vi "Create.vi"(8 "error in (no error)":errorcluster, 11 "Session in":refnum<class "Session.lvclass">) -> (0 "error out":errorcluster, 3 "Session out":refnum<class "Session.lvclass">)   [LabVIEW 2020, in "HTTP Server.lvlib" / "Session.lvclass"]
uses:
  Session.lvclass
  Session.lvclass/Session.ctl
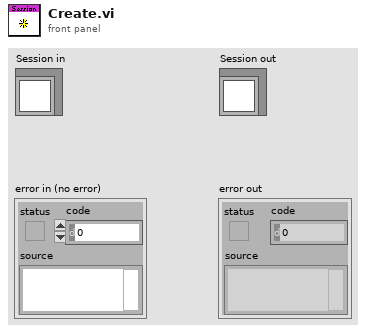
[diagram p1: front panel]
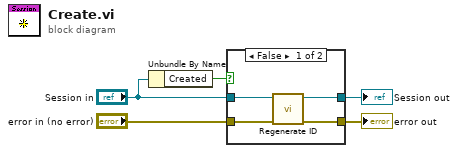
[diagram p0: block diagram]
diagram:
  n1 = Unbundle By Name("Session in") -> ("Created"=w1:bool)
  n2 = case shown="False" w1 {
    tunnel: [w9 w11] -> w5
    tunnel: "error in (no error)" -> [w8 w10]
    tunnel: [w7 w10] -> w3
    tunnel: "Session in" -> [w6 w11]
    frame False {
      n3 = call "Regenerate ID.vi"("error in (no error)"=w8, "Session in"=w6) -> ("error out"=w7:errorcluster, "Session out"=w9:refnum<class "Session.lvclass">)  [unwired: 6 in, 2 out]
    }
    frame True {
    }
  }
  "error out" <- w3
  "Session out" <- w5
